vi "QueueMany.vi"(9 "Playlist":string, 11 "Queue in":refnum<queue>) -> (3 "Queue out":refnum<queue>)   [LabVIEW 2016]
panel:
  out "Array":string[](array[string])
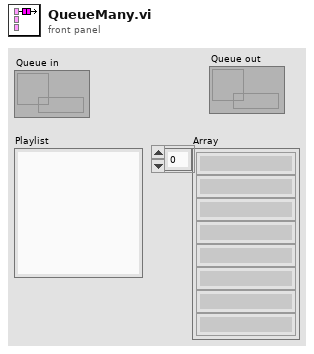
[diagram p1: front panel]
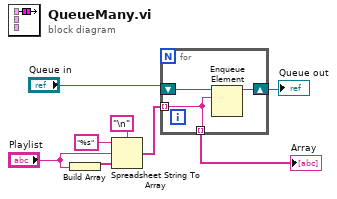
[diagram p0: block diagram]
diagram:
  n1 = Build Array("Playlist") -> (w1:string[])
  n2 = Spreadsheet String To Array(delimiter (Tab)="\n", format string="%s", spreadsheet string="Playlist", array type (2D Dbl)=w1) -> (array=w3:string[])
  n3 = for {
    shift-right: [w10] -> w8
    shift-left: "Queue in" -> [w11]
    tunnel: w3 -> [w9] mode=indexing
    tunnel: [w9] -> w6 mode=indexing
    n4 = Enqueue Element(queue=w11, element=w9) -> (queue out=w10:refnum<queue>)  [unwired: 2 in, 2 out]
  }
  "Queue out" <- w8
  "Array" <- w6
